vi "h5_write_3d_double_array.vi"(0 "h5 ref in":i32, 1 "dataset name":string, 5 "array":dbl[][][](array[numeric]), 7 "units (au)":string="au", 11 "error in (no error)":errorcluster, 12 "dim1 (index)":string="index", 13 "dim2 (index)":string="index", 14 "dim3 (index)":string="index") -> (4 "h5 ref out":i32, 15 "error out":errorcluster)   [LabVIEW 2015]
uses:
  <userlib>/_OpenG.lib/string/string.llb/To Camel Case (String)__ogtk.vi
  <vilib>/addons/h5labview2/base/lib_path.vi
  <vilib>/addons/h5labview2/base/H5Equery.vi
  <vilib>/addons/h5labview2/dataset/H5Dwrite.llb/H5Dwrite.xnode
  <vilib>/addons/h5labview2/attrib/H5Awrite.llb/H5Awrite.xnode
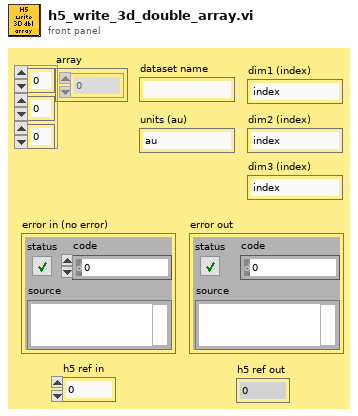
[diagram p1: front panel]
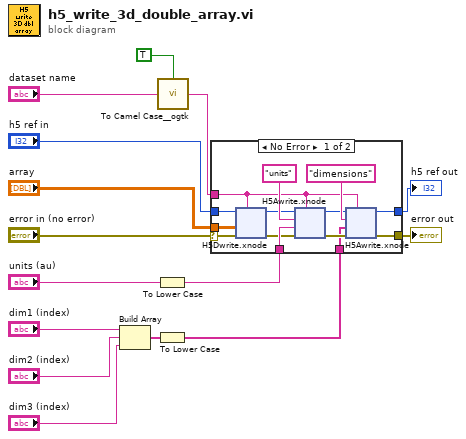
[diagram p0: block diagram]
diagram:
  n1 = Build Array("dim1 (index)", "dim2 (index)", "dim3 (index)") -> (w3:string[])
  n2 = To Lower Case(string="units (au)") -> (all lower case string=w4:string)
  n3 = To Lower Case(string=w3) -> (all lower case string=w2:string[])
  n4 = call-poly <userlib>:"To Camel Case__ogtk.vi"("string"="dataset name", "no change if no spaces? (F=No)"=TRUE) -> ("CamelCase string"=w6:string)
  n5 = case shown="No Error" "error in (no error)" {
    selector: "error in (no error)" -> [w17 w88]
    tunnel: "h5 ref in" -> [w29 w87]
    tunnel: w4 -> [w27 _]
    tunnel: "array" -> [w25 _]
    tunnel: w6 -> [w20 _]
    tunnel: [w19 w88] -> w13
    tunnel: [w18 w87] -> w12
    tunnel: w2 -> [w16 _]
    frame No Error {
      n6 = xnode "H5Dwrite.xnode"("dataset name"=w20, "error in (no error)"=w17, "data"=w25, "ref in"=w29) -> ("error out"=w24:errorcluster, "ref out"=w22:i32)  [unwired: 3 in, 1 out]
      n7 = xnode "H5Awrite.xnode"("object name"=w20, "error in (no error)"=w24, "data"=w27, "attrib name"="units", "ref in"=w22) -> ("error out"=w23:errorcluster, "ref out"=w21:i32)  [unwired: 2 in, 1 out]
      n8 = xnode "H5Awrite.xnode"("object name"=w20, "error in (no error)"=w23, "data"=w16, "attrib name"="dimensions", "ref in"=w21) -> ("error out"=w19:errorcluster, "ref out"=w18:i32)  [unwired: 2 in, 1 out]
    }
    frame Error {
    }
  }
  "error out" <- w13
  "h5 ref out" <- w12
